vi "Read Disconnection List.vi"(8 "error in (no error)":errorcluster, 11 "Switch Disconnect Message in":refnum<class "Switch Disconnect Message.lvclass">) -> (0 "error out":errorcluster, 2 "Disconnection List":string, 3 "Switch Disconnect Message out":refnum<class "Switch Disconnect Message.lvclass">)   [LabVIEW 2017, in "Messaging.lvlib" / "Switch Disconnect Message.lvclass"]
uses:
  Switch Disconnect Message.lvclass
  Switch Disconnect Message.lvclass/Switch Disconnect Message.ctl
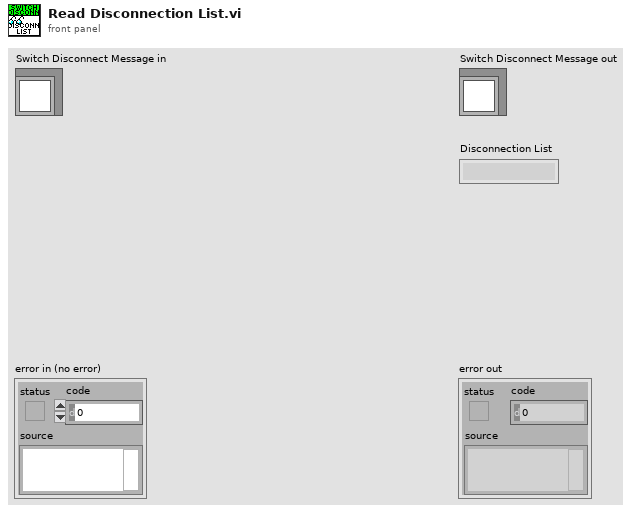
[diagram p1: front panel]
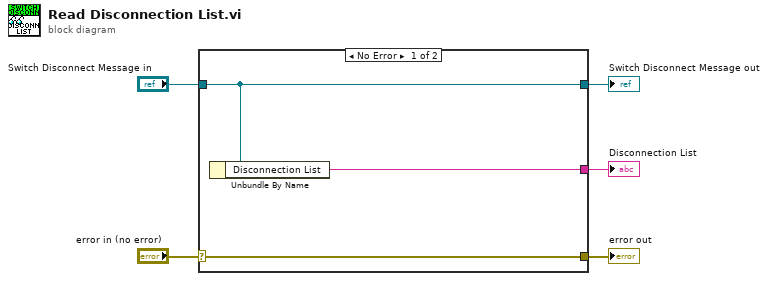
[diagram p0: block diagram]
diagram:
  n1 = case shown="No Error" "error in (no error)" {
    selector: "error in (no error)" -> [w8 w9]
    tunnel: [w8 w9] -> w4
    tunnel: [w7 w10] -> w2
    tunnel: "Switch Disconnect Message in" -> [w7 w10]
    tunnel: [w6 _] -> w1
    frame No Error {
      n2 = Unbundle By Name(w7) -> ("Disconnection List"=w6:string)
    }
    frame Error {
    }
  }
  "error out" <- w4
  "Switch Disconnect Message out" <- w2
  "Disconnection List" <- w1
